vi "Get Next Scan Angle.vi"(11 "scan angles in":T1) -> (2 "new angle":dbl, 3 "scan angles out":T1)   [LabVIEW 2017, in "NI_Robotics_Scan Angles.lvlib"]
uses:
  <vilib>/robotics/Utilities/Scan Angles/NI_Robotics_Scan Angles.lvlib
  <vilib>/robotics/Utilities/Scan Angles/Scan Angle Data.ctl
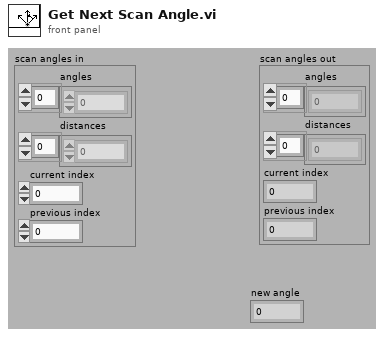
[diagram p1: front panel]
types:
  T1 = typedef "NI_Robotics_Scan Angles.lvlib/Scan Angle Data.ctl" = cluster{"angles":dbl[], "distances":dbl[], "current index":i32, "previous index":i32}
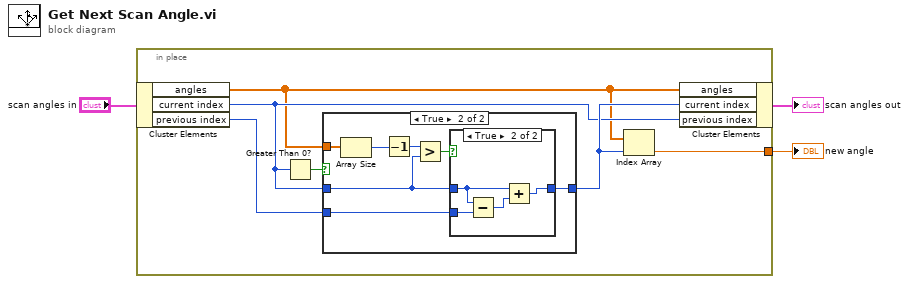
[diagram p0: block diagram]
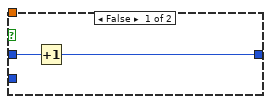
[diagram p2: hidden frame]
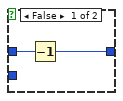
[diagram p3: hidden frame]
diagram:
  n1 = in-place {
    in-place-border: [w7] -> w1
    n2 = in-place-cluster #1("scan angles in") -> ("angles"=w5:dbl[], "current index"=w6:i32, "previous index"=w9:i32)
    n3 = Greater Than 0?(x=w6) -> (x > 0?=w4:bool)
    n4 = case shown="True" w4 {
      tunnel: w6 -> [w11 w15]
      tunnel: [w10 w14] -> w8
      tunnel: w5 -> [_ w18]
      tunnel: w9 -> [_ w13]
      frame False {
        n5 = Increment(x=w11) -> (x+1=w10:i32)
      }
      frame True {
        n6 = Array Size(array=w18) -> (size(s)=w17:i32)
        n7 = Decrement(x=w17) -> (x-1=w12:i32)
        n8 = Greater?(x=w12, y=w15) -> (0:w16:bool)
        n9 = case shown="True" w16 {
          tunnel: w15 -> [w20 w22]
          tunnel: [w19 w23] -> w14
          tunnel: w13 -> [_ w24]
          frame False {
            n10 = Decrement(x=w20) -> (x-1=w19:i32)
          }
          frame True {
            n11 = Subtract(x=w22, y=w24) -> (x-y=w21:i32)
            n12 = Add(x=w22, y=w21) -> (x+y=w23:i32)
          }
        }
      }
    }
    n13 = Index Array(array=w5, index=w8) -> (element=w7:dbl)
    n14 = in-place-cluster #1("angles"=w5, "current index"=w8, "previous index"=w6) -> (→"scan angles out":T1)
  }
  "new angle" <- w1
